vi "SaveToTblHist.vi"(8 "error in (no error)":errorcluster, 10 "OldTable (reset)":string[][](table), 11 "Table History ref":refnum<vi>) -> (0 "error out":errorcluster)   [LabVIEW 2013]
doc: "Add OldTable to the referred Table Undo (history) array. If TableHistory ref is not wired, no history is saved and currently there is no warning! CAUTION: Empty 'OldTable' signals that the history should be reset! This will be used for changes that cannot be undone like adding/removing devices. The default for OldTable is empty, causing it to reset if unwired."
uses:
  TypeDefs/TableHistory.ctl
  TypeDefs/TableArray.ctl
panel:
  out "Invalid ref?":bool
  out "reset?":bool
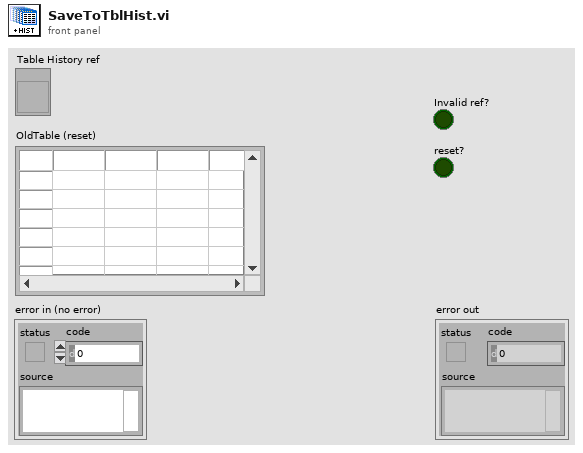
[diagram p1: front panel]
types:
  T1 = typedef "TableHistory.ctl" = cluster{"Undo pointer":i32, "OldTable Array":T2}
  T2 = typedef "TableArray.ctl" = string[]
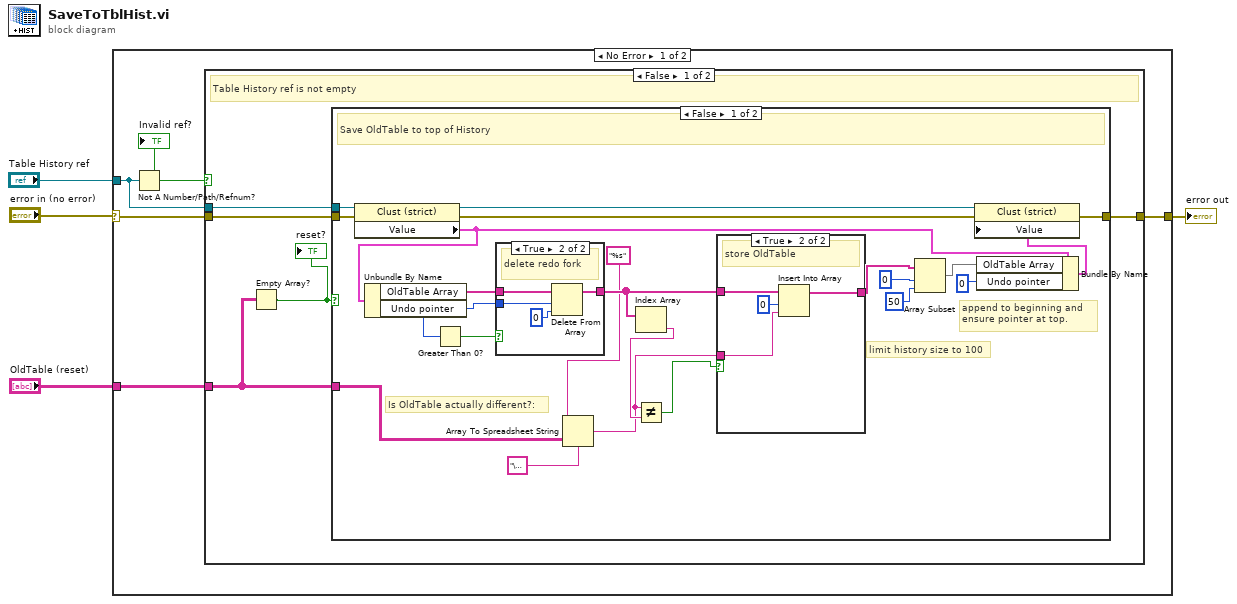
[diagram p0: block diagram]
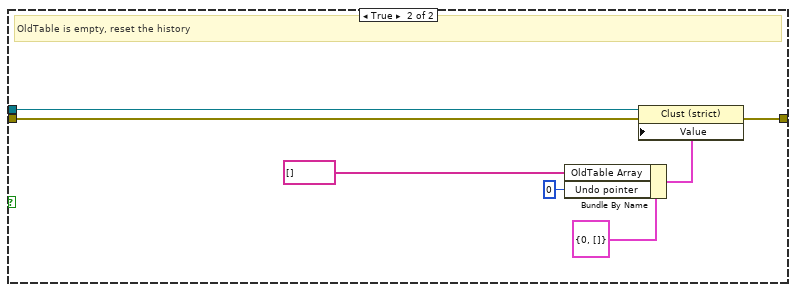
[diagram p4: hidden frame]
diagram:
  n1 = case shown="No Error" "error in (no error)" {
    selector: "error in (no error)" -> [w9 w55]
    tunnel: [w8 w55] -> w3
    tunnel: "OldTable (reset)" -> [w7 _]
    tunnel: "Table History ref" -> [w6 _]
    frame No Error {
      n2 = Not A Number/Path/Refnum?(number/path/refnum=w6) -> (NaN/Path/Refnum?=w5:bool)
      "Invalid ref?" <- w5
      n3 = case shown="False" w5 {
        tunnel: w9 -> [w14 w54]
        tunnel: [w13 w54] -> w8
        tunnel: w7 -> [w10 _]
        tunnel: w6 -> [w12 _]
        frame False {
          # "Table History ref is not empty"
          n4 = Empty Array?(array=w10) -> (empty?=w11:bool)
          "reset?" <- w11
          n5 = case shown="False" w11 {
            tunnel: w14 -> [w21 w52]
            tunnel: [w31 w51] -> w13
            tunnel: w12 -> [w22 w50]
            tunnel: w10 -> [w18 _]
            frame False {
              # "limit history size to 100"
              # "Is OldTable actually different?:"
              # "append to beginning and\nensure pointer at top."
              # "Save OldTable to top of History"
              n6 = property class="Clust (strict)"(reference=w22, error in=w21) -> (reference out=w33:refnum<vi>, error out=w32:errorcluster, "Value"=w23:T1)
              n7 = Unbundle By Name(w23) -> ("OldTable Array"=w36:T2, "Undo pointer"=w35:i32)
              n8 = Greater Than 0?(x=w35) -> (x > 0?=w34:bool)
              n9 = case shown="True" w34 {
                tunnel: w36 -> [w42 w46]
                tunnel: w35 -> [_ w45]
                tunnel: [w42 w43] -> w28
                frame False {
                  # "none for redo"
                }
                frame True {
                  # "delete redo fork"
                  n10 = Delete From Array(array=w46, length=w45, index=0) -> (array with subset deleted=w43:T2)  [unwired: 1 out]
                }
              }
              n11 = Array To Spreadsheet String(delimiter (Tab)="\u0000", array=w18, 3:"%s" ("format string")) -> (spreadsheet string=w15:string)
              n12 = Index Array(array=w28) -> (element=w19:string)  [unwired: 1 in]
              n13 = Not Equal?(x=w15, y=w19) -> (x != y?=w20:bool)
              n14 = case shown="True" w20 {
                tunnel: [w37 w41] -> w27
                tunnel: w28 -> [w37 w39]
                tunnel: w15 -> [_ w38]
                frame False {
                  # "already saved!"
                }
                frame True {
                  # "store OldTable"
                  n15 = Insert Into Array "Insert Into Array"(array=w39, index=0, new element=w38) -> (w41:T2)
                }
              }
              n16 = Array Subset(array=w27, index=0, length=50) -> (w24:T2)
              n17 = Bundle By Name(cluster=w23, "OldTable Array"=w24, "Undo pointer"=0) -> (w30:T1)
              n18 = property class="Clust (strict)"(reference=w33, error in=w32, "Value"=w30) -> (error out=w31:errorcluster)  [unwired: 1 out]
            }
            frame True {
              # "OldTable is empty, reset the history"
              n19 = Bundle By Name(cluster=T1 {"Undo pointer"=0, "OldTable Array"=[]} ("Value"), "OldTable Array"=T2 [], "Undo pointer"=0) -> (w53:T1)
              n20 = property class="Clust (strict)"(reference=w50, error in=w52, "Value"=w53) -> (error out=w51:errorcluster)  [unwired: 1 out]
            }
          }
        }
        frame True {
          # "possibly warn user here"
          # "no refnum to Table history (do nothing)"
        }
      }
    }
    frame Error {
    }
  }
  "error out" <- w3
